vi "GetEmptyTagValueList.vi"(8 "error in (no error)":errorcluster, 11 "dimension size (500)":i32=500) -> (0 "error out":errorcluster, 3 "Array":T1[](array[typedef]) {"Tag" format="%x" items=["NONE"=0, "Locked"=16, "SoftLock"=17, "KeyLock"=18, "Class_IV_Lock"=20, "Interlock"=24, "LaserMode"=32, "LDH_PulsePowerTable"=33, "TriggerMode"=48, "TriggerLevelRaw"=64, "TriggerLevelRawLoLimit"=65, "TriggerLevelRawHiLimit"=66, "TriggerLevel"=72, "TriggerLevelLoLimit"=73, "TriggerLevelHiLimit"=74, "FastGate"=80, "FastGateImp"=96, "SlowGate"=112, "TargetTempRaw"=144, "TargetTempRawLoLimit"=145, "TargetTempRawHiLimit"=146, "CurrentTempRaw"=148, "CaseTempRaw"=149, "TargetTemp"=152, "TargetTempLoLimit"=153, "TargetTempHiLimit"=154, "CurrentTemp"=156, "CaseTemp"=157, "TempScale"=159, "Frequency"=168, "FrequencyLoLimit"=169, "FrequencyHiLimit"=170, "PulsePowerRaw"=176, "PulsePowerRawLoLimit"=177, "PulsePowerRawHiLimit"=178, "PulsePowerPermille"=180, "PulseShape"=181, "PulsePower"=184, "PulsePowerLoLimit"=185, "PulsePowerHiLimit"=186, "PulsePowerNanowatt"=188, "PulsePowerVoltage"=190, "PulseEnergy"=191, "CwPowerRaw"=192, "CwPowerRawLoLimit"=193, "CwPowerRawHiLimit"=194, "CwPowerPermille"=196, "CwPower"=200, "CwPowerLoLimit"=201, "CwPowerHiLimit"=202, "CwPowerMicroWatt"=204, "BurstLen"=208, "BurstPeriod"=224, "LDH_Fan"=240, "UI_Exclusive"=256]})   [LabVIEW 2010]
doc: "Creates a new array of tag values"
uses:
  _lib/PDLM/pdlm_lib_x86_x64_UIThread.llb/PDLM_Tag.ctl
  _lib/PDLM/pdlm_lib_x86_x64_UIThread.llb/PDLM_TaggedValue.ctl
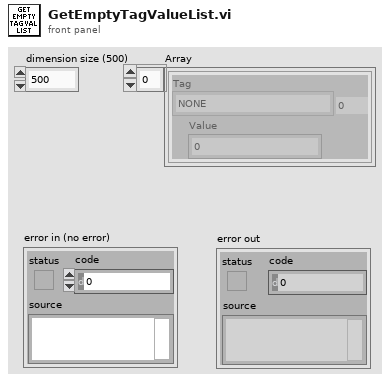
[diagram p1: front panel]
types:
  T1 = typedef "PDLM_TaggedValue.ctl" = cluster{"Tag":T2, "Value":u32}
  T2 = typedef "PDLM_Tag.ctl" = u32
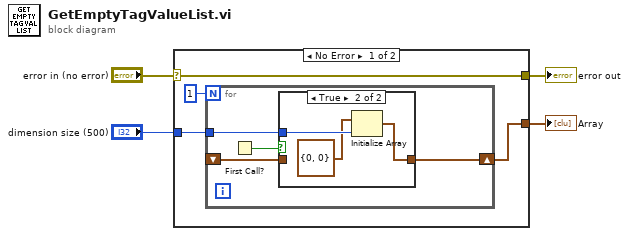
[diagram p0: block diagram]
diagram:
  n1 = case shown="No Error" "error in (no error)" {
    selector: "error in (no error)" -> [w6 w17]
    tunnel: [w8 _] -> w4
    tunnel: "dimension size (500)" -> [w7 _]
    tunnel: [w6 w17] -> w1
    frame No Error {
      n2 = for {
        N: 1 -> [_]
        tunnel: w7 -> [w11]
        shift-right: [w12] -> w8
        shift-left: _ -> [w9]
        n3 = First Call?() -> (First Call?: T/F=w10:bool)
        n4 = case shown="True" w10 {
          tunnel: [w13 w16] -> w12
          tunnel: w11 -> [_ w15]
          tunnel: w9 -> [w13 _]
          frame False {
          }
          frame True {
            n5 = Initialize Array(T1 {"Tag"=0, "Value"=0} ("TaggedValue"), w15) -> (w16:T1[])
          }
        }
      }
    }
    frame Error {
    }
  }
  "Array" <- w4
  "error out" <- w1
